vi "Magnet Set Field.vi"(6 "Field Strength":dbl, 7 "Polarity":bool, 8 "error in (no error)":errorcluster, 11 "VISA resource name in":refnum<visa-resource-name>) -> (0 "error out":errorcluster, 3 "VISA resource name out":refnum<visa-resource-name>)   [LabVIEW 2016, in "Hall Effect Library.lvlib"]
uses:
  Hall Effect Library.lvlib
  Global Variables/Instruments.vi
  Magnet Set Field (Manual).vi
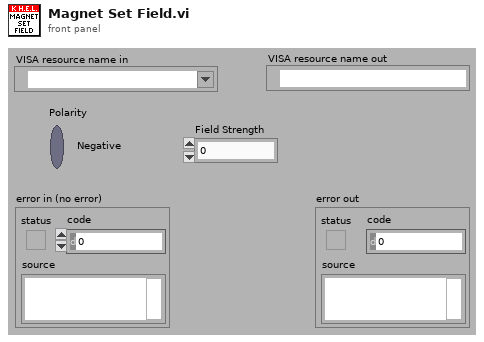
[diagram p1: front panel]
types:
  T1 = typedef "Hall Effect Library.lvlib/Magnets.ctl" = enum16{"Manual"}
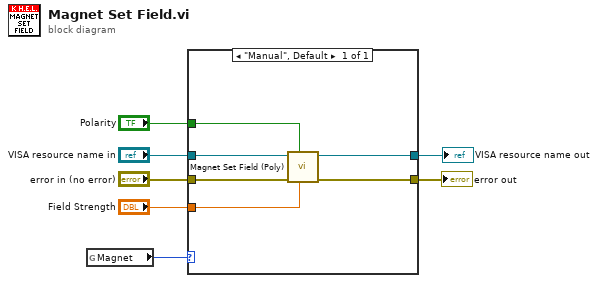
[diagram p0: block diagram]
diagram:
  n1 = global read "Instruments.vi" "Magnet"() -> (w7:T1)
  n2 = case shown="\"Manual\", Default" w7 {
    tunnel: "error in (no error)" -> [w13]
    tunnel: [w12] -> w5
    tunnel: [w11] -> w4
    tunnel: "VISA resource name in" -> [w10]
    tunnel: "Polarity" -> [w9]
    tunnel: "Field Strength" -> [w8]
    frame "Manual", Default {
      n3 = call-poly "Magnet Set Field (Poly).vi"("Field Strength"=w8, "Polarity"=w9, "error in (no error)"=w13, "VISA resource name in"=w10) -> ("error out"=w12:errorcluster, "VISA resource name out"=w11:refnum<visa-resource-name>)  [unwired: 6 out]
    }
  }
  "error out" <- w5
  "VISA resource name out" <- w4
